vi "relay.vi"() -> ()   [LabVIEW 2026]
uses:
  <vilib>/Instr/_visa.llb/VISA Configure Serial Port (Instr).vi
panel:
  in  "relay 2":bool
  in  "stop":bool
  in  "relay":bool
  in  "VISA resource name":refnum<visa-resource-name>
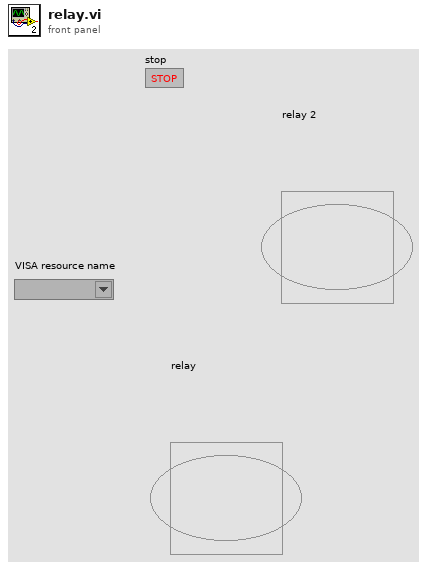
[diagram p1: front panel]
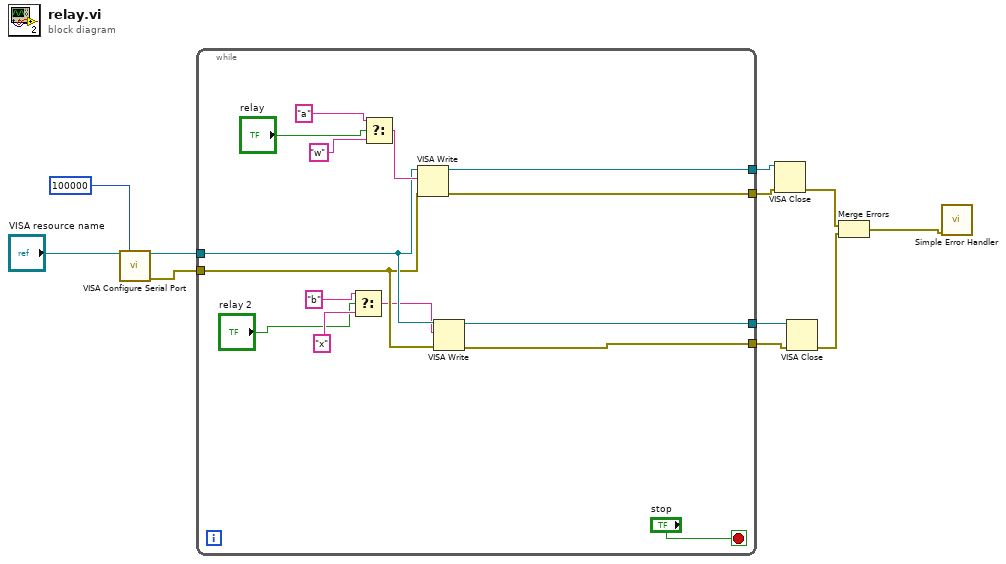
[diagram p0: block diagram]
diagram:
  n1 = call-poly "VISA Configure Serial Port"("VISA resource name"="VISA resource name", "timeout (10sec)"=u32 100000) -> ("VISA resource name out"=w9:refnum<visa-resource-name>, "error out"=w8:errorcluster)  [unwired: 12 in]
  n2 = while {
    tunnel: w9 -> [w25]
    tunnel: w8 -> [w24]
    tunnel: [w23] -> w7
    tunnel: [w22] -> w6
    tunnel: [w21] -> w5
    tunnel: [w20] -> w4
    stop <- "stop" stop-if-true
    n3 = Select(t="b", s="relay 2", f="x") -> (s? t:f=w16:string)
    n4 = Select(t="a", s="relay", f="w") -> (s? t:f=w26:string)
    n5 = VISA Write(VISA resource name=w25, write buffer=w26, error in (no error)=w24) -> (VISA resource name out=w23:refnum<visa-resource-name>, error out=w22:errorcluster)  [unwired: 1 out]
    n6 = VISA Write(VISA resource name=w25, write buffer=w16, error in (no error)=w24) -> (VISA resource name out=w21:refnum<visa-resource-name>, error out=w20:errorcluster)  [unwired: 1 out]
  }
  n7 = VISA Close(VISA resource name=w7, error in (no error)=w6) -> (error out=w3:errorcluster)
  n8 = VISA Close(VISA resource name=w5, error in (no error)=w4) -> (error out=w2:errorcluster)
  n9 = Merge Errors(w3, w2) -> (w1:errorcluster)
  n10 = call <vilib>:"Simple Error Handler.vi"("error in (no error)"=w1) -> ()  [unwired: 4 in, 5 out]
